vi "Plink GUI.vi"() -> ()   [LabVIEW 2013]
uses:
  Shared/GUI_Template/GUI_master/tcp_new_data_event.ctl
  Shared/GUI_Template/GUI_master/tcp new data cluster.ctl
  Non-General/BELLA/VIremote/VIremote.llb/VIremoteFunction.ctl
  <vilib>/Analysis/NI_AALBase.lvlib
panel:
  out "Device name":string
  in  "Refresh Button":bool
  in  "Select device":string(combo)="LB_PowerMeter"
  out "power":dbl=25.5 caption="Power (W)" min=0.0 max=300000000.0 format="%_4p"
  in  "stop":bool
  in  "Clear":bool
  out "XY Graph":cluster{dbl, dbl}[](graph)
  out "sigma":dbl=25.5 caption="Sigma" min=0.0 max=300000000.0 format="%_4p"
  out "mean":dbl=25.5 caption="Mean" min=0.0 max=300000000.0 format="%_4p"
  in  "error IO":errorcluster
  in  "Energy Mode::1":enum16{"off", "on"}(ring) caption="Energy Mode"
  in  "triggerlevel::1":dbl=0.5 caption="Trig Level" min=0.0 max=100.0 format="%_4f"
  out "Wavelength::1":i32 caption="Wavelength" min=0 max=5000
  out "tcp data event":T1
  out "error IO 2":errorcluster
  out "GUIdevice 1":string="BELLA_TEA_PowerMeter"
  in  "insert tag":bool=TRUE
  in  "Reading::1":dbl=0.5 caption="Power (W)" min=0.0 max=50000.0 format="%_4p"
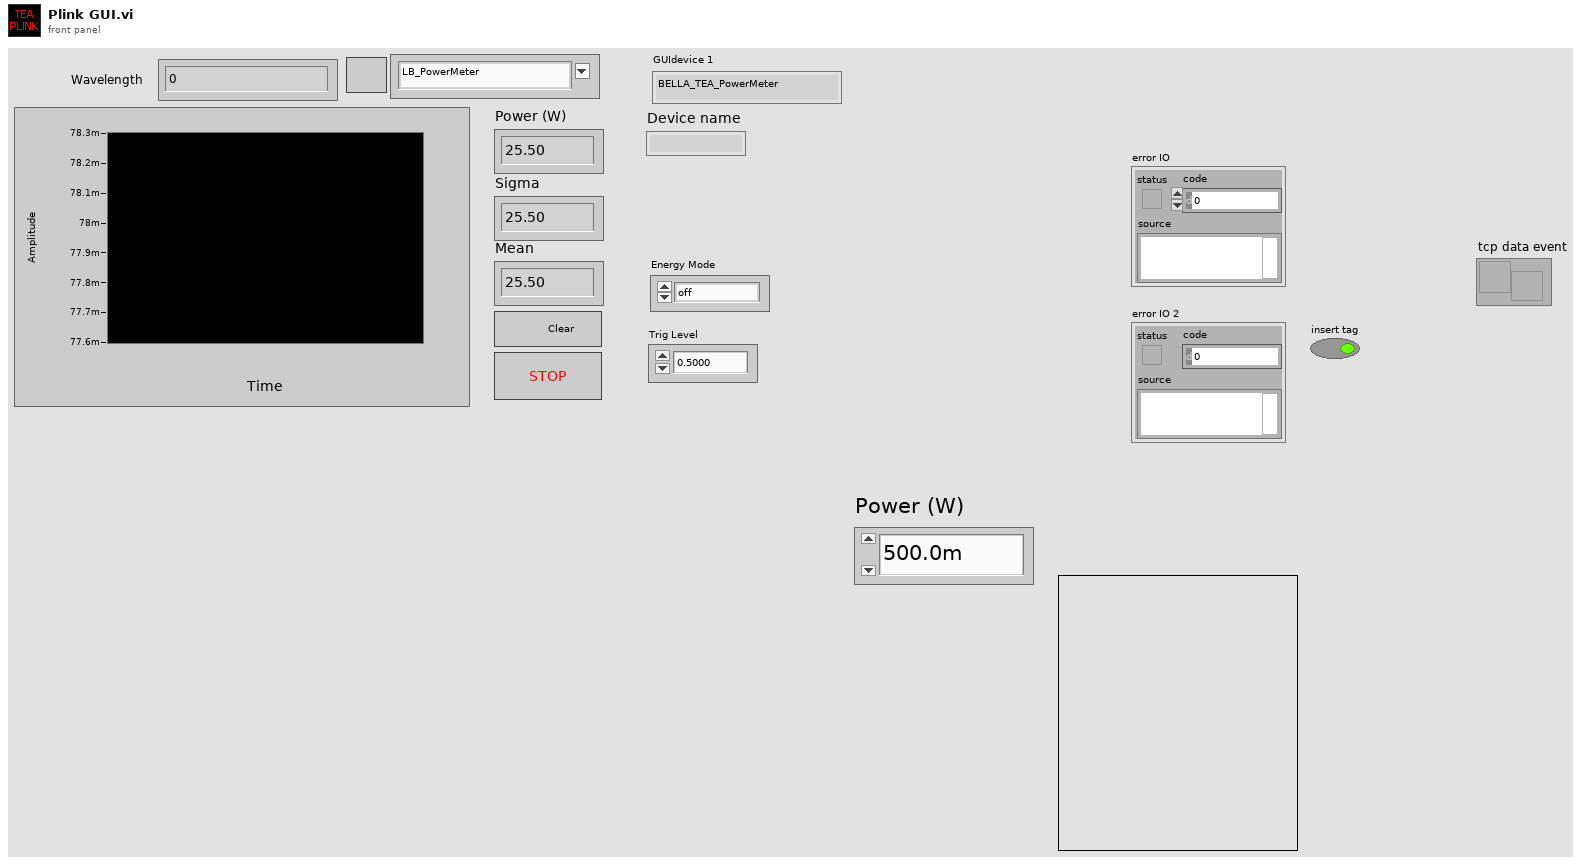
[diagram p1: front panel]
types:
  T1 = typedef "tcp_new_data_event.ctl" = refnum<user-event>
  T2 = typedef "tcp new data cluster.ctl" = cluster{"EventEnum":enum16{"new data", "connection status update"}, "Device name":string}
  T3 = typedef "VIremoteFunction.ctl" = enum16{"Do nothing", "Stop controller", "Close this connection", "Show info panel", "Set VI to control", "Set Accelerometer freq (Hz)", "Show Alert message", "Start Sound Input", "Stop Sound Input", "Set Volume (0-100)", "Set sound output Speaker", "Set sound output Receiver", "Play Sound", "Repeat Sound", "Stop Sound", "Pause Sound", "Resume Sound", "Set panel width of caller (320 or 480)", "Set Panel Size to Portrait", "Set Panel Size to Landscape", "Set Panel Size as Current Orientation", "Allow all UI Orientations", "Send user notification", "Disable Scrolling", "Normal Scrolling", "Page Scrolling", "Set Scroll Offset", "Page Indicator Position"}
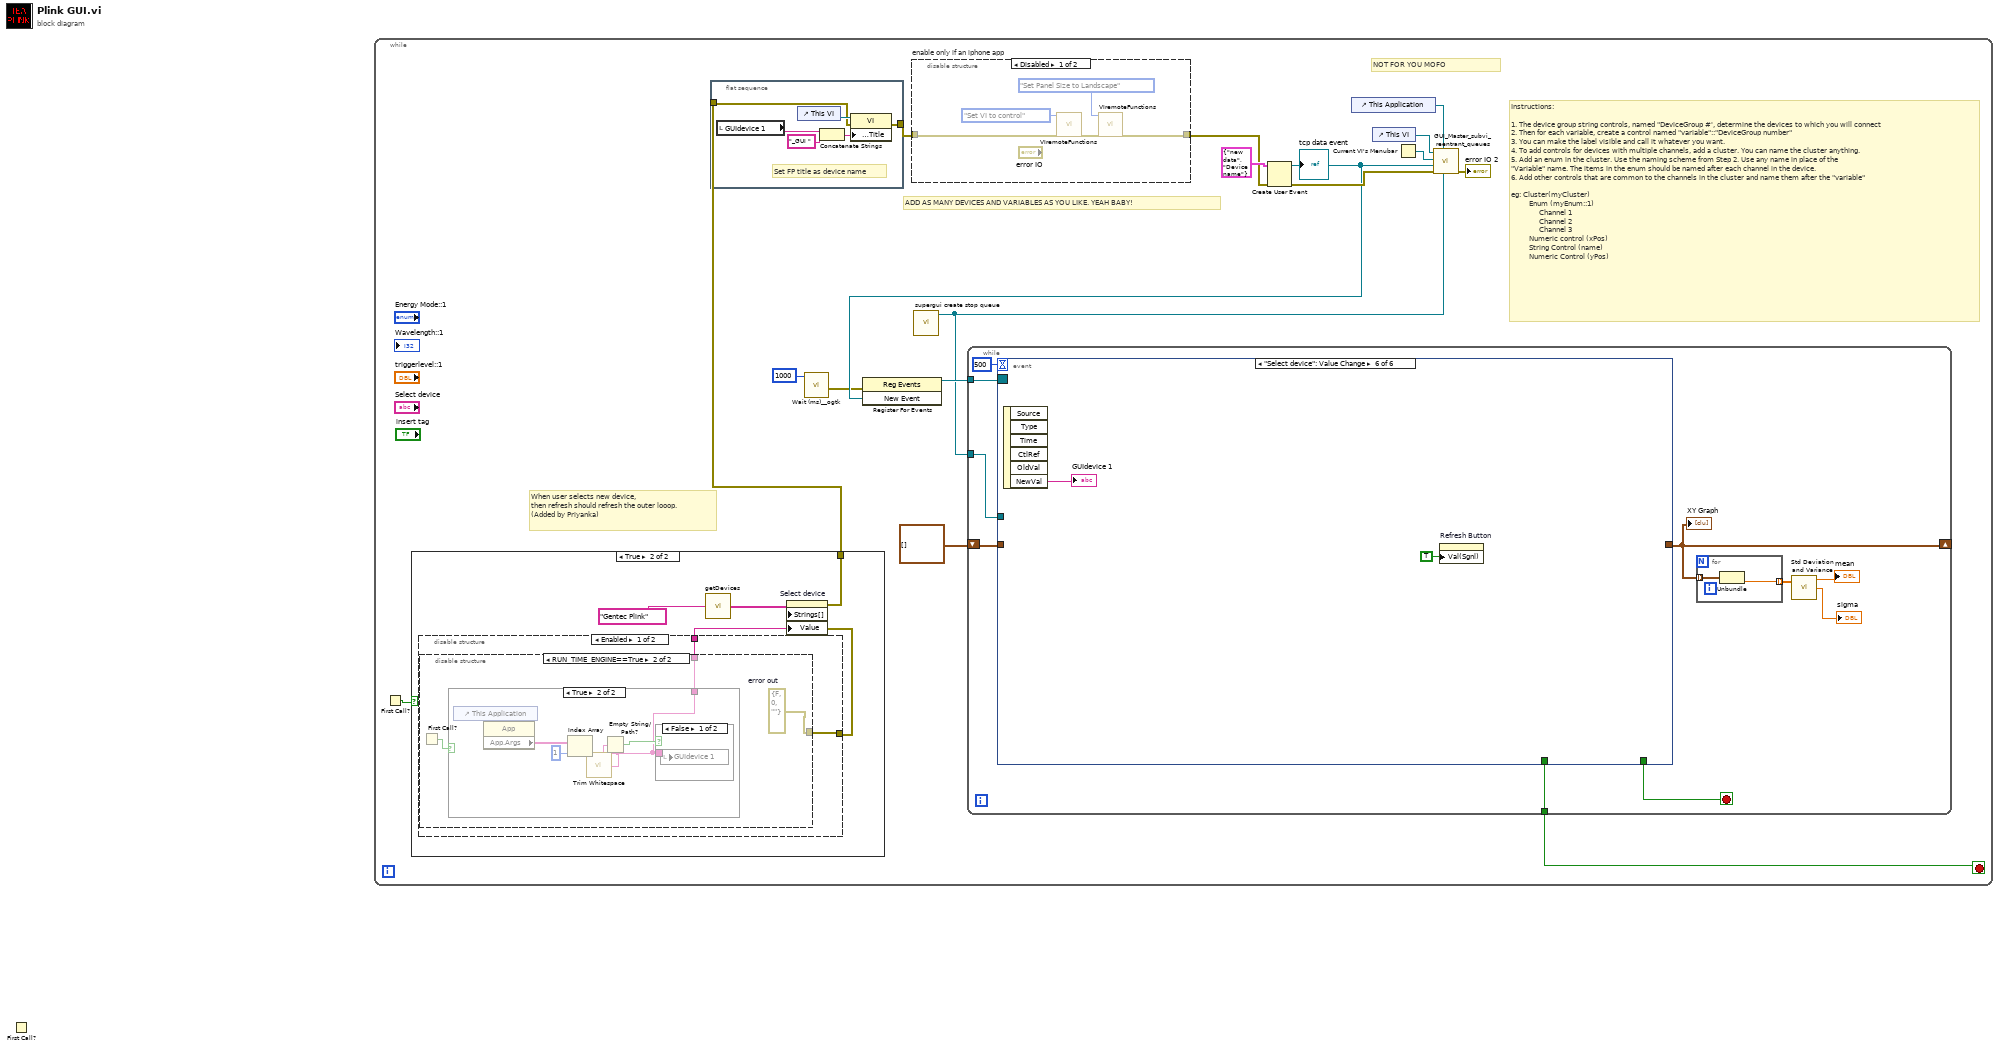
[diagram p0: block diagram]
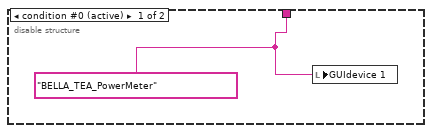
[diagram p3: hidden frame]
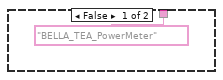
[diagram p4: hidden frame]
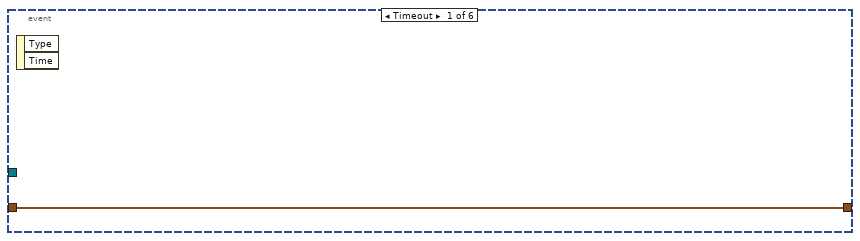
[diagram p7: hidden frame]
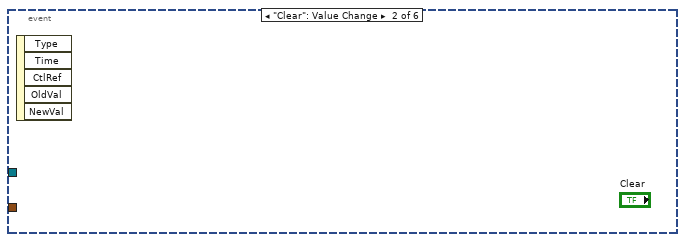
[diagram p8: hidden frame]
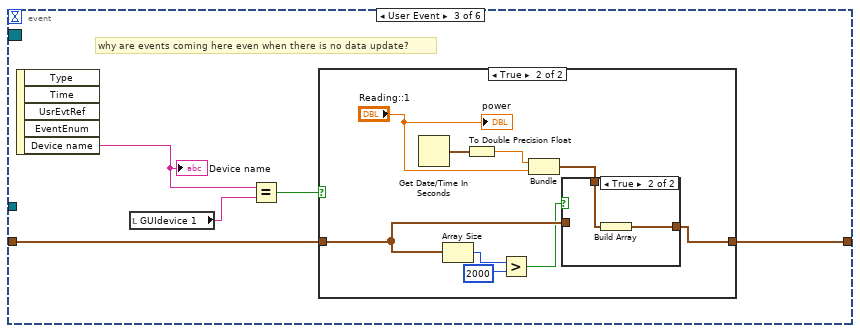
[diagram p9: hidden frame]
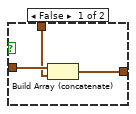
[diagram p11: hidden frame]
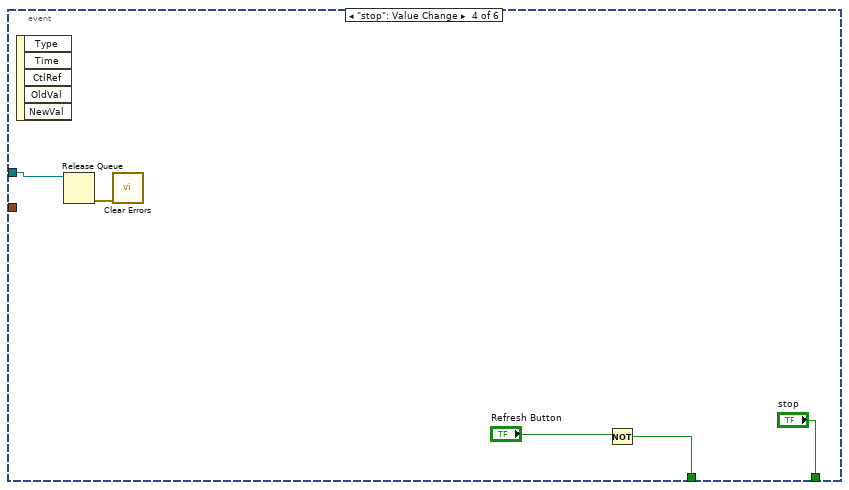
[diagram p12: hidden frame]
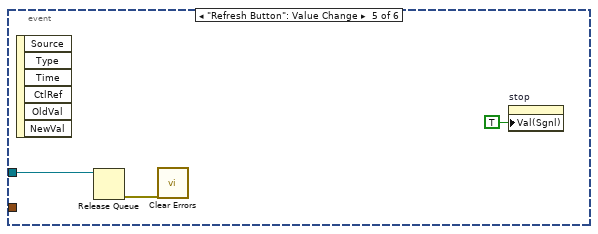
[diagram p13: hidden frame]
diagram:
  n1 = First Call?() -> ()  [unwired: 1 out]
  n2 = while {
    stop <- w4 stop-if-true
    # "When user selects new device,\nthen refresh should refresh the outer looop.\n(Added by Priyanka)"
    # "Instructions:\n\n1. The device group string controls, named \"DeviceGroup #', determine the devices to which you will connect\n2. Then for each variable, create a control named \"variable\"::\"DeviceGroup number\"\n3. You can make the label visible and call it whatever you want.\n4. To add controls for devices with multiple channels, add a cluster. You can name the cluster anything.\n5. Add an enum in the cluster. Use the naming scheme from Step 2. Use any name in place of the \n\"Variable\" name. The items in the enum should be named after each channel in the device. \n6. Add other controls that are common to the channels in the cluster and name them after the \"variable\"\n\neg: Cluster(myCluster)\n         Enum (myEnum::1)\n              Channel 1 \n              Channel 2\n              Channel 3\n         Numeric control (xPos)\n         String Control (name)\n         Numeric Control (yPos)"
    # "ADD AS MANY DEVICES AND VARIABLES AS YOU LIKE. YEAH BABY!"
    # "NOT FOR YOU MOFO"
    n3 = First Call?() -> (First Call?: T/F=w5:bool)
    n4 = case shown="True" w5 {
      tunnel: [_ w26] -> w3
      frame False {
      }
      frame True {
        n5 = disable-structure shown="Enabled" {
          disable-tunnel: [w30 _] -> w25
          disable-tunnel: [w29 _] -> w24
          frame Enabled {
            n6 = disable-structure shown="RUN_TIME_ENGINE==True" {
              disable-tunnel: [_ w34] -> w30
              disable-tunnel: [w31 w32] -> w29
              frame condition #0 (active) {
                w31 = "BELLA_TEA_PowerMeter" ("trimmed string")
                n7 = local write "GUIdevice 1"(w31) -> ()
              }
              frame condition #1 {
                w34 = errorcluster {"status"=FALSE, "code"=0, "source"=""}  # error out
                n8 = First Call?() -> (First Call?: T/F=w33:bool)
                n9 = case shown="True" w33 {
                  tunnel: ["BELLA_TEA_PowerMeter" ("trimmed string") w36] -> w32
                  frame False {
                  }
                  frame True {
                    n10 = control-ref of="This Application"() -> (w38:refnum<vi>)
                    n11 = property class="App"(reference=w38) -> ("App.Args"=w41:string[])  [unwired: 1 in, 2 out]
                    n12 = Index Array(array=w41, index=1) -> (element=w39:string)
                    n13 = call <vilib>:"Trim Whitespace.vi"("string"=w39) -> ("trimmed string"=w36:string)  [unwired: 1 in]
                    n14 = Empty String/Path?(string/path=w36) -> (empty?=w40:bool)
                    n15 = case shown="False" w40 {
                      tunnel: w36 -> [w42 _]
                      frame False {
                        n16 = local write "GUIdevice 1"(w42) -> ()
                      }
                      frame True {
                      }
                    }
                  }
                }
              }
            }
          }
          frame Disabled {
          }
        }
        n17 = call "getDevices.vi"("Device Class"="Gentec Plink") -> ("All Devices"=w27:string[])
        n18 = property on="Select device" class="CmbBox"(error in=w25, "Strings[]"=w27, "Value"=w24) -> (error out=w26:errorcluster)  [unwired: 1 in, 1 out]
      }
    }
    n19 = flat-sequence {
      tunnel: [w20] -> w2
      tunnel: w3 -> [w19]
      frame #0 {
        # "Set FP title as device name"
        n20 = local read "GUIdevice 1"() -> (w18:string)
        n21 = control-ref of="This VI"() -> (w23:refnum<vi>)
        n22 = Concatenate Strings(w18, "_GUI ") -> (w22:string)
        n23 = property class="VI"(reference=w23, error in=w19, "Front Panel.Title"=w22) -> (error out=w20:errorcluster)  [unwired: 1 out]
      }
    }
    n24 = call <userlib>:"Wait (ms)__ogtk.vi"("milliseconds to wait"=u32 1000) -> ("error out"=w6:errorcluster)  [unwired: 9 in, 1 out]
    n25 = disable-structure "enable only if an iphone app" shown="Disabled" {
      disable-tunnel: [w87 w91] -> w12
      disable-tunnel: w2 -> [w86 w91]
      frame Disabled {
        n26 = call "VIremoteFunctions.vi"("error in (no error)"=w86, "Function"=VIremoteFunction."Set VI to control") -> ("error out"=w88:errorcluster)  [unwired: 4 in, 5 out]
        n27 = call "VIremoteFunctions.vi"("error in (no error)"=w88, "Function"=VIremoteFunction."Set Panel Size to Landscape") -> ("error out"=w87:errorcluster)  [unwired: 4 in, 5 out]
      }
      frame Enabled {
      }
    }
    n28 = call "supergui create stop queue.vi"() -> ("STOP Queue out"=w1:refnum<queue>)  [unwired: 11 in]
    n29 = Create User Event(user event datatype=T2 {"EventEnum"=enum."new data", "Device name"="Device name"} ("New Event"), error in=w12) -> (user event=w9:refnum<user-event>, error out=w13:errorcluster)
    "tcp data event" <- w9
    n30 = register-events(error in=w6, w9) -> (reference out=w10:refnum<event-registration>)  [unwired: 1 in, 1 out]
    n31 = while {
      tunnel: w10 -> [w52]
      shift-right: [w48] -> _
      shift-left: cluster{dbl, "data::1":dbl}[] [] -> [w49]
      tunnel: [w44] -> w4
      tunnel: w1 -> [w43]
      stop <- w50 stop-if-true
      n32 = event shown="[5] \"Select device\": Value Change" {
        selector: w52 -> [_ _ _ _ _ _]
        dyn-events: _ -> [_ _ _ _ _ _]
        timeout: 500 -> [_ _ _ _ _ _]
        tunnel: [_ _ _ "stop" _ _] -> w50
        tunnel: w49 -> [w55 _ w60 _ _ _]
        tunnel: [w55 _ w59 _ _ _] -> w48
        tunnel: [_ _ _ w78 _ _] -> w44
        tunnel: w43 -> [_ _ _ w77 w82 _]
        event Timeout {
          n33 = event-data() -> ()  [unwired: 1 in, 2 out]
        }
        event "Clear": Value Change {
          n34 = event-data() -> ()  [unwired: 1 in, 5 out]
        }
        event User Event {
          # "why are events coming here even when there is no data update?"
          n35 = event-data() -> ("Device name"=w58:string)  [unwired: 1 in, 4 out]
          "Device name" <- w58
          n36 = local read "GUIdevice 1"() -> (w57:string)
          n37 = Equal?(x=w58, y=w57) -> (x = y?=w56:bool)
          n38 = case shown="True" w56 {
            tunnel: w60 -> [w61 w70]
            tunnel: [w61 w66] -> w59
            frame False {
            }
            frame True {
              n39 = Get Date/Time In Seconds() -> (seconds since 1Jan1904=w64:timestamp)
              n40 = Array Size(array=w70) -> (size(s)=w69:i32)
              n41 = To Double Precision Float(number=w64) -> (double precision float=w65:dbl)
              n42 = Greater?(x=w69, y=2000) -> (0:w67:bool)
              n43 = Bundle(w65, "Reading::1"="Reading::1") -> (w63:cluster{dbl, "Reading::1":dbl})  [unwired: 1 in]
              n44 = case shown="True" w67 {
                tunnel: w70 -> [w73 _]
                tunnel: [w72 w75] -> w66
                tunnel: w63 -> [w71 w74]
                frame False {
                  n45 = Build Array (concatenate)(w73, w71) -> (w72:cluster{dbl, "Reading::1":dbl}[])
                }
                frame True {
                  n46 = Build Array(w74) -> (w75:cluster{dbl, "Reading::1":dbl}[])
                }
              }
              "power" <- "Reading::1"
            }
          }
        }
        event "stop": Value Change {
          n47 = event-data() -> ()  [unwired: 1 in, 5 out]
          n48 = Release Queue(queue=w77) -> (error out=w76:errorcluster)  [unwired: 2 in, 2 out]
          n49 = call <vilib>:"Clear Errors.vi"("error in (no error)"=w76) -> ()  [unwired: 6 in, 1 out]
          n50 = Not(x="Refresh Button") -> (.not. x?=w78:bool)
        }
        event "Refresh Button": Value Change {
          n51 = event-data() -> ()  [unwired: 1 in, 6 out]
          n52 = Release Queue(queue=w82) -> (error out=w81:errorcluster)  [unwired: 2 in, 2 out]
          n53 = call <vilib>:"Clear Errors.vi"("error in (no error)"=w81) -> ()  [unwired: 6 in, 1 out]
          n54 = property on="stop" class="Bool (strict)"("Val(Sgnl)"=TRUE ("Value (Signaling)")) -> ()  [unwired: 2 in, 2 out]
        }
        event "Select device": Value Change {
          n55 = event-data() -> ("NewVal"=→"GUIdevice 1":string)  [unwired: 1 in, 5 out]
          n56 = property on="Refresh Button" class="Bool (strict)"("Val(Sgnl)"=TRUE ("Value (Signaling)")) -> ()  [unwired: 2 in, 2 out]
        }
      }
      "XY Graph" <- w48
      n57 = for {
        tunnel: w48 -> [w54] mode=indexing
        tunnel: [w53] -> w47 mode=indexing
        n58 = Unbundle(w54) -> ("Reading::1"=w53:dbl)  [unwired: 1 out]
      }
      n59 = call <vilib>:"Std Deviation and Variance.vi"("X"=w47) -> ("mean"=→"mean":dbl, "standard deviation"=→"sigma":dbl)  [unwired: 1 in, 1 out]
    }
    n60 = control-ref of="This Application"() -> (w7:refnum<vi>)
    n61 = control-ref of="This VI"() -> (w16:refnum<vi>)
    n62 = Current VI's Menubar() -> (w15:refnum<k9>)
    n63 = call "GUI_Master_subvi_reentrant_queues.vi"("STOP Queue in"=w1, "This Application"=w7, "error in (no error)"=w13, "tcp data event"=w9, "Caller menu reference"=w15, "Caller VI ref"=w16) -> ("error out"=→"error IO 2":errorcluster)  [unwired: 5 in]
  }
